vi "Runge Kutta Check.vi"(8 "F(X,t)":string[](array[string]), 9 "X":string[](array[string]), 10 "time":string, 11 "X(0)":dbl[](array[numeric]) format="%.2f") -> (0 "system OK":bool, 1 "error text":string[](array[string]), 2 "error":i32[](array[numeric]), 3 "error message":string, 4 "result":dbl[][](array[numeric]), 5 "table":i32[][][](array[numeric]))   [LabVIEW 2020, in "NI_Gmath.lvlib"]
uses:
  <vilib>/gmath/NI_Gmath.lvlib
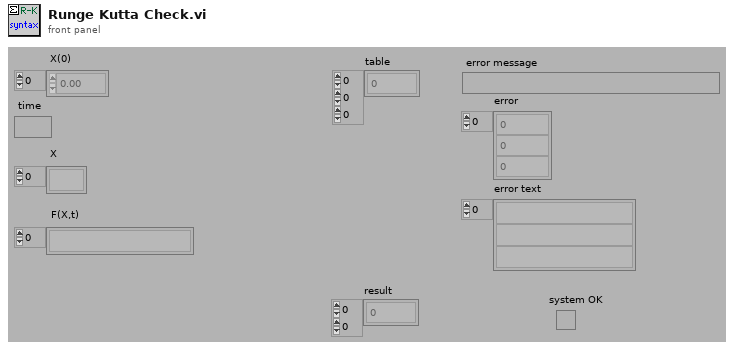
[diagram p1: front panel]
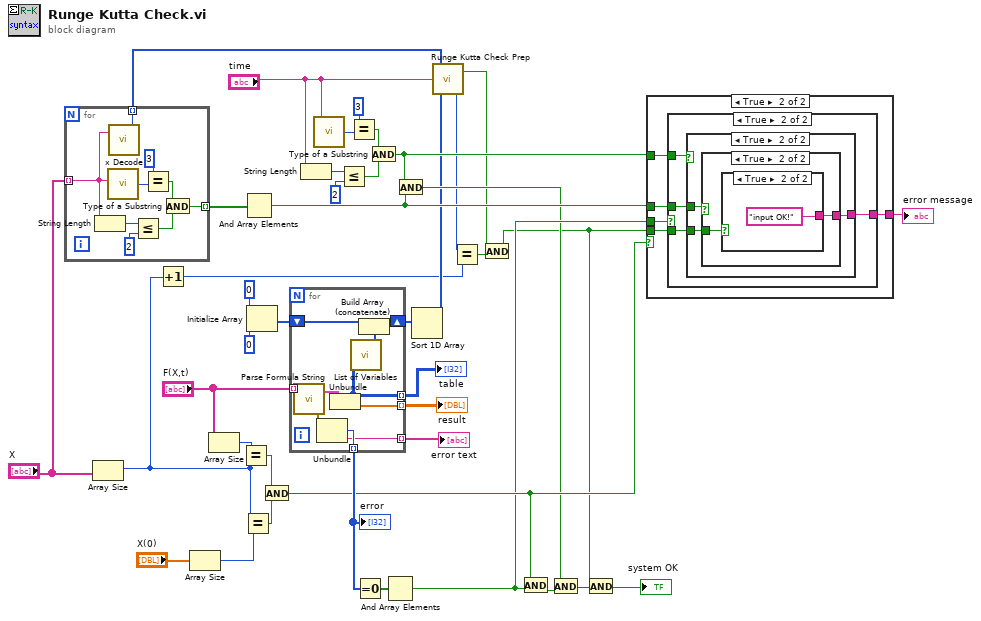
[diagram p0: block diagram]
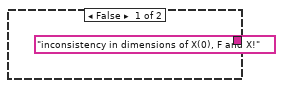
[diagram p2: hidden frame]
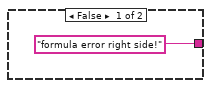
[diagram p3: hidden frame]
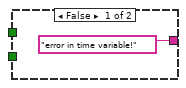
[diagram p4: hidden frame]
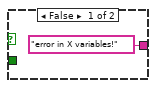
[diagram p5: hidden frame]
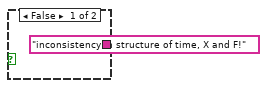
[diagram p6: hidden frame]
diagram:
  n1 = for {
    tunnel: "X" -> [w43] mode=indexing
    tunnel: [w44] -> w22 mode=indexing
    tunnel: [w42] -> w13 mode=indexing
    n2 = String Length(string=w43) -> (length=w45:i32)
    n3 = call <vilib>:"Type of a Substring.VI"("item"=w43) -> ("type"=w47:i32)
    n4 = call <vilib>:"x Decode.vi"("x string"=w43) -> ("number"=w42:i32)  [unwired: 1 in, 1 out]
    n5 = Less Or Equal?(x=w45, y=2) -> (x <= y?=w49:bool)
    n6 = Equal?(x=3, y=w47) -> (x = y?=w50:bool)
    n7 = And(x=w50, y=w49) -> (x .and. y?=w44:bool)
  }
  n8 = Array Size(array="X") -> (size(s)=w12:i32)
  n9 = Increment(x=w12) -> (x+1=w11:i32)
  n10 = Array Size(array="X(0)") -> (size(s)=w35:i32)
  n11 = Array Size(array="F(X,t)") -> (size(s)=w36:i32)
  n12 = Equal?(x=w36, y=w12) -> (x = y?=w33:bool)
  n13 = Equal?(x=w12, y=w35) -> (x = y?=w34:bool)
  n14 = And Array Elements(Boolean array=w22) -> (logical AND=w20:bool)
  n15 = Initialize Array(0, 0) -> (w16:i32[])
  n16 = And(x=w33, y=w34) -> (x .and. y?=w32:bool)
  n17 = for {
    tunnel: [w55] -> w40 mode=indexing
    tunnel: [w53] -> w39 mode=indexing
    tunnel: [w52] -> w38 mode=indexing
    tunnel: "F(X,t)" -> [w57] mode=indexing
    shift-right: [w59] -> w15
    shift-left: w16 -> [w60]
    tunnel: [w51] -> w1 mode=indexing
    n18 = call <vilib>:"Parse Formula String.vi"("formula"=w57) -> ("error out"=w56:errorcluster, "Parsed Formula"=w54:cluster{"Table":i32[][], "Y Values":dbl[]})  [unwired: 1 in]
    n19 = Unbundle(w56) -> ("code"=w55:i32, "source"=w51:string)  [unwired: 1 out]
    n20 = Unbundle(w54) -> ("Table"=w53:i32[][], "Y Values"=w52:dbl[])
    n21 = call <vilib>:"List of Variables.vi"("Table"=w53) -> ("List of variables"=w58:i32[])
    n22 = Build Array (concatenate)(w60, w58) -> (w59:i32[])
  }
  "error" <- w40
  "error text" <- w1
  "result" <- w38
  "table" <- w39
  n23 = String Length(string="time") -> (length=w29:i32)
  n24 = call <vilib>:"Type of a Substring.VI"("item"="time") -> ("type"=w27:i32)
  n25 = Less Or Equal?(x=w29, y=2) -> (x <= y?=w25:bool)
  n26 = Equal?(x=3, y=w27) -> (x = y?=w24:bool)
  n27 = Equal To 0?(x=w40) -> (x = 0?=w41:bool[])
  n28 = And(x=w24, y=w25) -> (x .and. y?=w21:bool)
  n29 = And Array Elements(Boolean array=w41) -> (logical AND=w30:bool)
  n30 = And(x=w21, y=w20) -> (x .and. y?=w19:bool)
  n31 = Sort 1D Array(array=w15) -> (sorted array=w14:i32[])
  n32 = call <vilib>:"Runge Kutta Check Prep.vi"("F(X,t) coded"=w14, "time"="time", "X coded"=w13) -> ("number of X variables"=w10:i32, "variables correct?"=w8:bool)
  n33 = Equal?(x=w10, y=w11) -> (x = y?=w9:bool)
  n34 = And(x=w8, y=w9) -> (x .and. y?=w7:bool)
  n35 = And(x=w32, y=w30) -> (x .and. y?=w23:bool)
  n36 = And(x=w19, y=w23) -> (x .and. y?=w6:bool)
  n37 = And(x=w7, y=w6) -> (x .and. y?=→"system OK":bool)
  n38 = case shown="True" w32 {
    tunnel: ["inconsistency in dimensions of X(0), F and X!" w66] -> w31
    tunnel: w30 -> [_ w65]
    tunnel: w20 -> [_ w64]
    tunnel: w21 -> [_ w63]
    tunnel: w7 -> [_ w62]
    frame False {
    }
    frame True {
      n39 = case shown="True" w65 {
        tunnel: ["formula error right side!" w71] -> w66
        tunnel: w64 -> [_ w70]
        tunnel: w63 -> [_ w69]
        tunnel: w62 -> [_ w68]
        frame False {
        }
        frame True {
          n40 = case shown="True" w69 {
            tunnel: ["error in time variable!" w75] -> w71
            tunnel: w70 -> [_ w74]
            tunnel: w68 -> [_ w73]
            frame False {
            }
            frame True {
              n41 = case shown="True" w74 {
                tunnel: ["error in X variables!" w78] -> w75
                tunnel: w73 -> [_ w77]
                frame False {
                }
                frame True {
                  n42 = case shown="True" w77 {
                    tunnel: ["inconsistency in structure of time, X and F!" "input OK!"] -> w78
                    frame False {
                    }
                    frame True {
                    }
                  }
                }
              }
            }
          }
        }
      }
    }
  }
  "error message" <- w31
